vi "10.vi"() -> ()   [LabVIEW 2017, in "ErrorStructureDrawer-Tests.lvlib"]
uses:
  ErrorStructureDrawer-Tests.lvlib
panel:
  out "refnum out":refnum<file>
  in  "file path (use dialog)":path
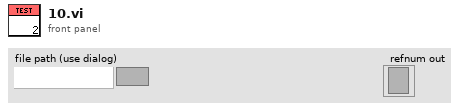
[diagram p1: front panel]
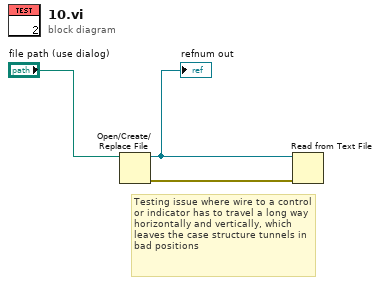
[diagram p0: block diagram]
diagram:
  # "Testing issue where wire to a control or indicator has to travel a long way horizontally and vertically, which leaves the case structure tunnels in bad positions"
  n1 = Open/Create/Replace File(file path (use dialog)="file path (use dialog)") -> (refnum out=w1:refnum<file>, error out=w2:errorcluster)  [unwired: 5 in, 1 out]
  "refnum out" <- w1
  n2 = Read from Text File(file (use dialog)=w1, error in=w2) -> ()  [unwired: 2 in, 4 out]
